vi "WriteElement.vi"(8 "error in (no error)":errorcluster, 10 "dvr element":T1, 11 "name":string) -> (0 "error out":errorcluster, 1 "initialize":bool, 3 "replaced dvr":u32)   [LabVIEW 2017, in "DVRBuffer.lvlib"]
uses:
  <vilib>/addons/InsightCM/Devices/Shared/Common/DVRBuffer/DVRBuffer.lvlib
  <vilib>/addons/InsightCM/Devices/Shared/Common/DVRBuffer/controls/DVRElement.ctl
  <vilib>/addons/InsightCM/Devices/Shared/Common/DVRBuffer/controls/DVRBuffer.ctl
  <vilib>/addons/PointValueMap/subVIs/Point_Read_variant.vi
  <vilib>/addons/PointValueMap/subVIs/Point_Write_variant.vi
  <vilib>/addons/PointValueMap/PointValueMap.lvlib
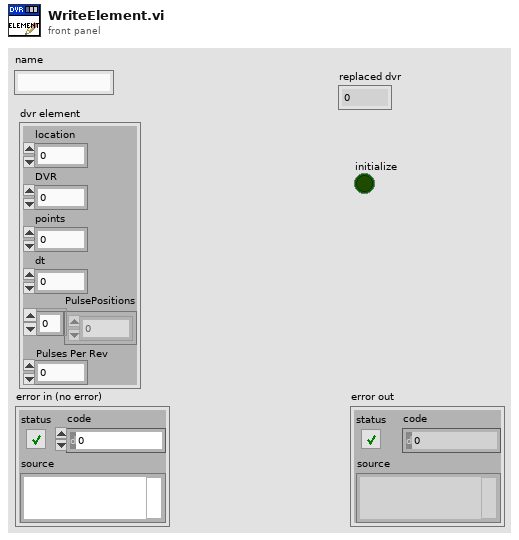
[diagram p1: front panel]
types:
  T1 = typedef "DVRBuffer.lvlib/DVRElement.ctl" = cluster{"location":u32, "DVR":u32, "points":i32, "dt":dbl, "PulsePositions":dbl[], "Pulses Per Rev":dbl}
  T2 = typedef "PointValueMap.lvlib/PointMap.ctl" = refnum<data-value>
  T3 = typedef "DVRBuffer.lvlib/DVRBuffer.ctl" = cluster{"buffer":T1[], "write ptr index":i32, "last block":u32, "buffer size":u32}
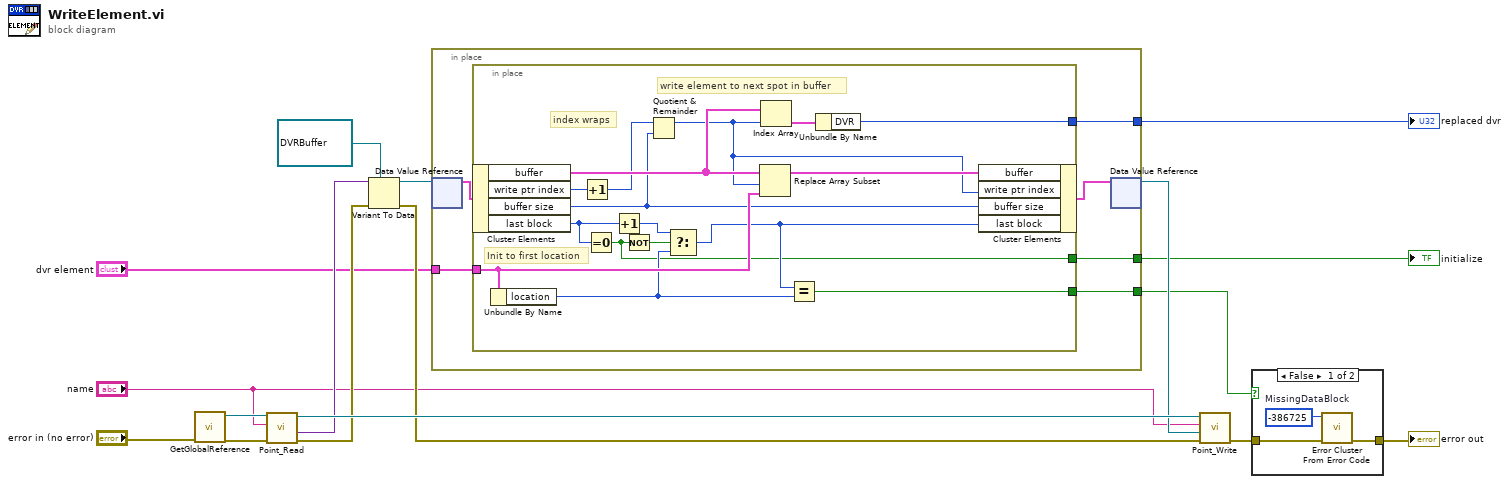
[diagram p0: block diagram]
diagram:
  n1 = call <vilib>:"GetGlobalReference.vi"("error in (no error)"="error in (no error)") -> ("error out"=w16:errorcluster, "reference"=w11:T2)  [unwired: 9 in]
  n2 = call-poly <vilib>:"Point_Read.vi"("Error In"=w16, "Tag"="name", "Map"=w11) -> ("Error Out"=w10:errorcluster, "Value"=w9:variant, "Map Out"=w14:T2)  [unwired: 3 in, 3 out]
  n3 = Variant To Data(error in=w10, type=refnum<data-value> refnum ("data value reference"), Variant=w9) -> (data=w15:refnum<data-value>, error out=w13:errorcluster)
  n4 = in-place {
    in-place-border: [w21] -> w6
    in-place-border: [w20] -> w3
    in-place-border: "dvr element" -> [w19]
    in-place-border: [w18] -> w1
    n5 = in-place-dvr #1(w15) -> (w23:T3)  [unwired: 1 out]
    n6 = in-place {
      in-place-border: [w36] -> w21
      in-place-border: [w35] -> w20
      in-place-border: w19 -> [w34]
      in-place-border: [w25] -> w18
      # "Init to first location"
      # "index wraps"
      # "write element to next spot in buffer"
      n7 = in-place-cluster #2(w23) -> ("buffer"=w38:T1[], "write ptr index"=w33:i32, "buffer size"=w32:u32, "last block"=w29:u32)
      n8 = Unbundle By Name(w34) -> ("location"=w28:u32)
      n9 = Increment(x=w33) -> (x+1=w31:i32)
      n10 = Equal To 0?(x=w29) -> (x = 0?=w25:bool)
      n11 = Increment(x=w29) -> (x+1=w27:u32)
      n12 = Not(x=w25) -> (.not. x?=w24:bool)
      n13 = Quotient & Remainder(x=w31, y=w32) -> (x-y*floor(x/y)=w30:u32)  [unwired: 1 out]
      n14 = Select(t=w27, s=w24, f=w28) -> (s? t:f=w26:u32)
      n15 = Replace Array Subset(array=w38, new element=w34, index=w30) -> (w39:T1[])
      n16 = Index Array(array=w38, index=w30) -> (element=w37:T1)
      n17 = Equal?(x=w26, y=w28) -> (x = y?=w35:bool)
      n18 = Unbundle By Name(w37) -> ("DVR"=w36:u32)
      n19 = in-place-cluster #2("buffer"=w39, "write ptr index"=w30, "buffer size"=w32, "last block"=w26) -> (w22:T3)
    }
    n20 = in-place-dvr #1(w22) -> (w12:refnum<data-value>)  [unwired: 1 out]
  }
  "replaced dvr" <- w6
  "initialize" <- w1
  n21 = call-poly <vilib>:"Point_Write.vi"("Error In"=w13, "Value"=w12, "Tag"="name", "Map"=w14) -> ("Error Out"=w5:errorcluster)  [unwired: 6 in, 1 out]
  n22 = case shown="False" w3 {
    tunnel: [w40 w43] -> w4
    tunnel: w5 -> [w41 w43]
    frame False {
      w42 = -386725  # MissingDataBlock
      n23 = call <vilib>:"Error Cluster From Error Code.vi"("error in (no error)"=w41, "error code (0)"=w42) -> ("error out"=w40:errorcluster)  [unwired: 7 in]
    }
    frame True {
    }
  }
  "error out" <- w4
